vi "myRIO v1.0 Shutdown PWM.vi"(8 "error in (no error)":errorcluster, 10 "Channel":T1, 11 "myRIO Ref In":T2) -> (0 "error out":errorcluster, 3 "myRIO Ref Out":T2)   [LabVIEW 2021]
uses:
  <vilib>/myRIO/Common/Instrument Driver Framework/Utilities/typedefs/myRIO v1.0 Reference.ctl
  <vilib>/myRIO/Common/Instrument Driver Framework/Utilities/typedefs/Generic FPGA Reference.ctl
  <vilib>/myRIO/Common/Instrument Driver Framework/myRIO v1.0/PWM/typedefs/PWM Channels Enum.ctl
  <vilib>/myRIO/Common/Instrument Driver Framework/myRIO v1.0/PWM/typedefs/PWM Channels FPGA Reference.ctl
  <vilib>/rvi/errors/niLvFpgaAdjustHostInterfaceError.vi
  <vilib>/rvi/interface/nirviReadWriteControl/nirviReadWriteControl.xnode
  NiFpgaLv.dll
  <vilib>/rvi/interface/Simulation/niFpgaSimulationCallBeginRW.vi
panel:
  # "This VI turns off the specified PWM channel and zeroes out all of its registers."
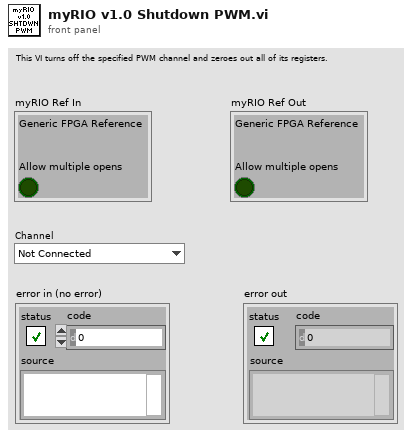
[diagram p1: front panel]
types:
  T1 = typedef "PWM Channels Enum.ctl" = enum16{"Not Connected", "C/PWM0", "C/PWM1", "A/PWM0", "A/PWM1", "A/PWM2", "A/PWM3", "A/PWM4", "A/PWM5", "A/PWM6", "A/PWM7", "A/PWM8", "A/PWM9", "A/PWM10", "A/PWM11", "A/PWM12", "A/PWM13", "A/PWM14", "A/PWM15", "A/PWM16", "A/PWM17", "A/PWM18", "A/PWM19", "B/PWM0", "B/PWM1", "B/PWM2", "B/PWM3", "B/PWM4", "B/PWM5", "B/PWM6", "B/PWM7", "B/PWM8", "B/PWM9", "B/PWM10", "B/PWM11", "B/PWM12", "B/PWM13", "B/PWM14", "B/PWM15", "B/PWM16", "B/PWM17", "B/PWM18", "B/PWM19", "PWM/PWM0", "PWM/PWM1", "PWM/PWM2", "PWM/PWM3", "PWM/PWM4", "PWM/PWM5", "PWM/PWM6", "PWM/PWM7", "PWM/PWM8", "PWM/PWM9"}
  T2 = typedef "myRIO v1.0 Reference.ctl" = cluster{"Generic FPGA Reference":T3, "Allow multiple opens":bool}
  T3 = typedef "Generic FPGA Reference.ctl" = refnum<k20>
  T4 = typedef "PWM Channels FPGA Reference.ctl" = refnum<k20>
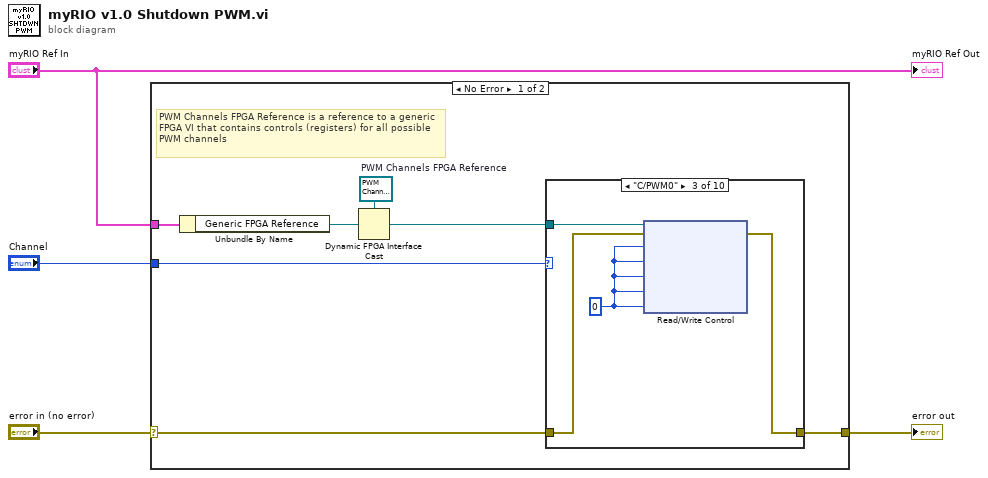
[diagram p0: block diagram]
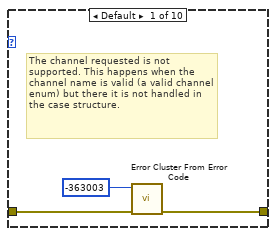
[diagram p2: hidden frame]
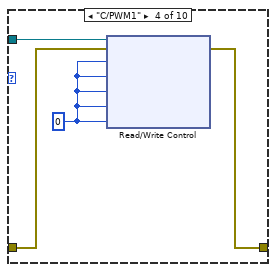
[diagram p4: hidden frame]
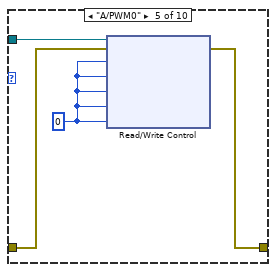
[diagram p5: hidden frame]
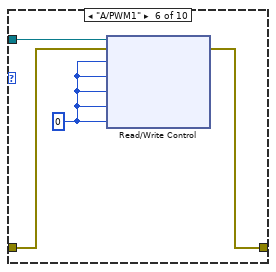
[diagram p6: hidden frame]
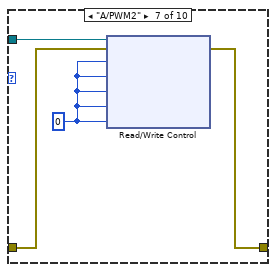
[diagram p7: hidden frame]
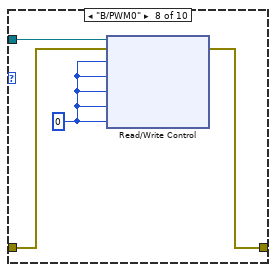
[diagram p8: hidden frame]
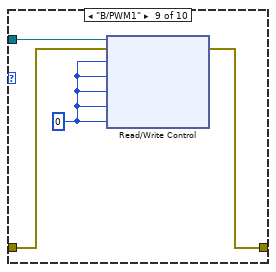
[diagram p9: hidden frame]
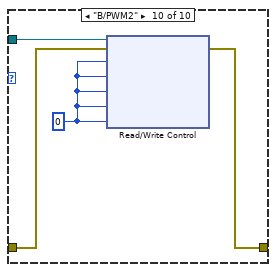
[diagram p10: hidden frame]
diagram:
  n1 = case shown="No Error" "error in (no error)" {
    selector: "error in (no error)" -> [w6 w48]
    tunnel: "myRIO Ref In" -> [w9 _]
    tunnel: [w8 w48] -> w3
    tunnel: "Channel" -> [w7 _]
    frame No Error {
      w11 = T4 refnum  # PWM Channels FPGA Reference
      # "PWM Channels FPGA Reference is a reference to a generic FPGA VI that contains controls (registers) for all possible PWM channels"
      n2 = Unbundle By Name(w9) -> ("Generic FPGA Reference"=w5:T3)
      n3 = Dynamic FPGA Interface Cast(Session In=w11, Type=w5) -> (Session Out=w10:T4)
      n4 = case shown="\"C/PWM0\"" w7 {
        tunnel: w6 -> [w12 w15 w19 w23 w27 w31 w35 w39 w43 w47]
        tunnel: [w13 w15 w18 w22 w26 w30 w34 w38 w42 w46] -> w8
        tunnel: w10 -> [_ _ w17 w21 w25 w29 w33 w37 w41 w45]
        frame Default {
          # "The channel requested is not supported. This happens when the channel name is valid (a valid channel enum) but there it is not handled in the case structure."
          n5 = call <vilib>:"Error Cluster From Error Code.vi"("error in (no error)"=w12, "error code (0)"=-363003) -> ("error out"=w13:errorcluster)  [unwired: 7 in]
        }
        frame "Not Connected" {
        }
        frame "C/PWM0" {
          w16 = u16 0 ("PWM.C_0.MAX")
          n6 = xnode "Read/Write Control"("FPGA VI Reference In"=w17, "error in"=w19, "PWM.C_0.CS"=w16, "PWM.C_0.CNFG"=w16, "PWM.C_0.CNTR"=w16, "PWM.C_0.CMP"=w16, "PWM.C_0.MAX"=w16) -> ("error out"=w18:errorcluster)  [unwired: 1 out]
        }
        frame "C/PWM1" {
          w20 = u16 0 ("PWM.C_0.MAX")
          n7 = xnode "Read/Write Control"("FPGA VI Reference In"=w21, "error in"=w23, "PWM.C_1.CS"=w20, "PWM.C_1.CNFG"=w20, "PWM.C_1.CNTR"=w20, "PWM.C_1.CMP"=w20, "PWM.C_1.MAX"=w20) -> ("error out"=w22:errorcluster)  [unwired: 1 out]
        }
        frame "A/PWM0" {
          w24 = u16 0 ("PWM.C_0.MAX")
          n8 = xnode "Read/Write Control"("FPGA VI Reference In"=w25, "error in"=w27, "PWM.A_0.CS"=w24, "PWM.A_0.CNFG"=w24, "PWM.A_0.CNTR"=w24, "PWM.A_0.CMP"=w24, "PWM.A_0.MAX"=w24) -> ("error out"=w26:errorcluster)  [unwired: 1 out]
        }
        frame "A/PWM1" {
          w28 = u16 0 ("PWM.C_0.MAX")
          n9 = xnode "Read/Write Control"("FPGA VI Reference In"=w29, "error in"=w31, "PWM.A_1.CS"=w28, "PWM.A_1.CNFG"=w28, "PWM.A_1.CNTR"=w28, "PWM.A_1.CMP"=w28, "PWM.A_1.MAX"=w28) -> ("error out"=w30:errorcluster)  [unwired: 1 out]
        }
        frame "A/PWM2" {
          w32 = u16 0 ("PWM.C_0.MAX")
          n10 = xnode "Read/Write Control"("FPGA VI Reference In"=w33, "error in"=w35, "PWM.A_2.CS"=w32, "PWM.A_2.CNFG"=w32, "PWM.A_2.CNTR"=w32, "PWM.A_2.CMP"=w32, "PWM.A_2.MAX"=w32) -> ("error out"=w34:errorcluster)  [unwired: 1 out]
        }
        frame "B/PWM0" {
          w36 = u16 0 ("PWM.C_0.MAX")
          n11 = xnode "Read/Write Control"("FPGA VI Reference In"=w37, "error in"=w39, "PWM.B_0.CS"=w36, "PWM.B_0.CNFG"=w36, "PWM.B_0.CNTR"=w36, "PWM.B_0.CMP"=w36, "PWM.B_0.MAX"=w36) -> ("error out"=w38:errorcluster)  [unwired: 1 out]
        }
        frame "B/PWM1" {
          w40 = u16 0 ("PWM.C_0.MAX")
          n12 = xnode "Read/Write Control"("FPGA VI Reference In"=w41, "error in"=w43, "PWM.B_1.CS"=w40, "PWM.B_1.CNFG"=w40, "PWM.B_1.CNTR"=w40, "PWM.B_1.CMP"=w40, "PWM.B_1.MAX"=w40) -> ("error out"=w42:errorcluster)  [unwired: 1 out]
        }
        frame "B/PWM2" {
          w44 = u16 0 ("PWM.C_0.MAX")
          n13 = xnode "Read/Write Control"("FPGA VI Reference In"=w45, "error in"=w47, "PWM.B_2.CS"=w44, "PWM.B_2.CNFG"=w44, "PWM.B_2.CNTR"=w44, "PWM.B_2.CMP"=w44, "PWM.B_2.MAX"=w44) -> ("error out"=w46:errorcluster)  [unwired: 1 out]
        }
      }
    }
    frame Error {
      # "Nothing to do since there was an incoming error."
    }
  }
  "error out" <- w3
  "myRIO Ref Out" <- "myRIO Ref In"
